vi "saturation.vi"(7 "uMax":sgl, 10 "signal in":sgl) -> (2 "signal out":sgl)   [LabVIEW 2017]
uses:
  <vilib>/Platform/TimedLoop/XDataNode/timing_clust.ctl
  <vilib>/Platform/TimedLoop/XDataNode/nitl_modes.ctl
  <vilib>/Platform/TimedLoop/XDataNode/wakeup.ctl
  floating_point_toolkit/PolymorphicSubVis/Negate 00.vi
  <vilib>/rvi/Emulation/niFpgaSctlEmulationGetInTimedLoop.vi
  <vilib>/rvi/Emulation/niFpgaEmulationReportErrorSimple.vi
  <vilib>/rvi/Emulation/niFpgaGetClockAttributes.vi
  <vilib>/rvi/Emulation/niFpgaCriticalErrorInLSC.vi
  <vilib>/Platform/TimedLoop/XDataNode/XDataNode.xnode
  <vilib>/Platform/TimedLoop/XDataNode/XDNodeRunTimeDep.lvlib
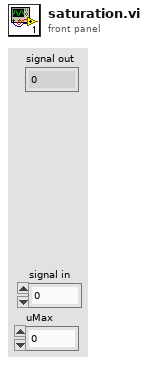
[diagram p1: front panel]
types:
  T1 = typedef "XDNodeRunTimeDep.lvlib/timing_clust.ctl" = cluster{"Expected End [f-1]":u64, "Actual End [f-1]":u64, "Finished Late? [f-1]":bool, "Expected End [i-1]":u64, "Actual End [i-1]":u64, "Finished Late? [i-1]":bool, "Expected Start [i]":u64, "Actual Start [i]":u64, "Expected Start [f]":u64, "Actual Start [f]":u64, "Source Name":string, "Structure Name":string, "Period":i64, "Deadline":i64, "Offset":i64, "Start":i64, "Priority":i32, "Timeout":i32, "Mode":T2, "Wakeup Reason":T3, "Error":errorcluster, "Source Type":string, "Secondary Source Type":string, "Global End Time":u64, "Global Start Time":u64, "Frame Duration":u64, "Iteration Duration":u64, "Assigned CPU":i32, "I/O Scan Engine Mode":u32}
  T2 = typedef "XDNodeRunTimeDep.lvlib/nitl_modes.ctl" = enum32{"No Change", "Process missed periods, maintain original phase", "Discard missed periods, maintain original phase", "Process missed periods, ignore original phase", "Discard missed periods, ignore original phase"}
  T3 = typedef "XDNodeRunTimeDep.lvlib/wakeup.ctl" = enum32{"Normal", "Aborted", "Asynchronous wakeup", "Timing source error", "Timed loop error", "Timeout"}
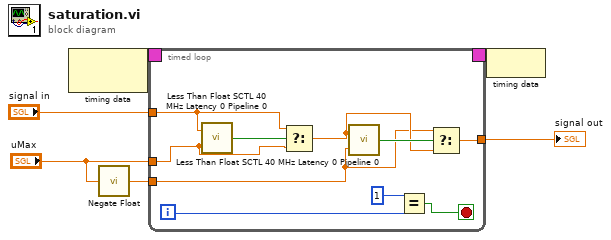
[diagram p0: block diagram]
diagram:
  n1 = node-c288() -> (w4:T1)  [unwired: 1 in]
  n2 = call-poly "Negate Float.vi"("x"="uMax") -> ("-x"=w2:sgl)
  n3 = timed-loop {
    timing: w4 -> [_]
    timing-out: [_] -> w3
    tunnel: "uMax" -> [w8]
    tunnel: "signal in" -> [w14]
    tunnel: [w13] -> w5
    tunnel: w2 -> [w7]
    i -> [w10]
    stop <- w11 stop-if-true
    n4 = call "Less Than Float SCTL 40 MHz Latency 0 Pipeline 0.vi"("y"=w8, "x"=w14) -> ("x < y?"=w16:bool)
    n5 = Select(t=w14, s=w16, f=w8) -> (s? t:f=w12:sgl)
    n6 = call "Less Than Float SCTL 40 MHz Latency 0 Pipeline 0.vi"("y"=w7, "x"=w12) -> ("x < y?"=w15:bool)
    n7 = Equal?(x=i16 1, y=w10) -> (x = y?=w11:bool)
    n8 = Select(t=w7, s=w15, f=w12) -> (s? t:f=w13:sgl)
  }
  "signal out" <- w5
  n9 = node-c288(w3) -> ()
